vi "Read Status.vi"(8 "Error In":errorcluster, 11 "Writer In":refnum<class "Writer.lvclass">) -> (0 "Error Out":errorcluster, 2 "Status":T1, 3 "Writer Out":refnum<class "Writer.lvclass">)   [LabVIEW 2018, in "Toolkit.lvlib" / "Writer.lvclass"]
doc: "Gets the latest status of the internal encoder."
uses:
  Writer.lvclass
  Controls/Status.ctl
  Writer.lvclass/Writer.ctl
  Toolkit.lvlib
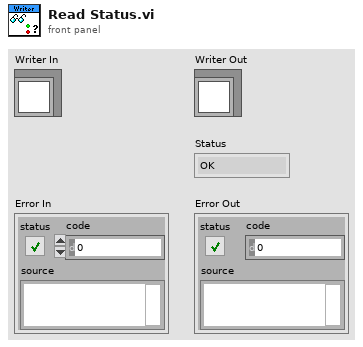
[diagram p1: front panel]
types:
  T1 = typedef "Toolkit.lvlib/Status.ctl" = enum32{"OK", "Out of Memory", "Null Value", "Encoder", "Decoder"}
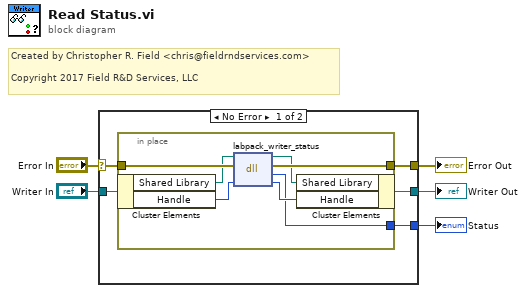
[diagram p0: block diagram]
diagram:
  # "Created by Christopher R. Field <chris@fieldrndservices.com>\n\nCopyright 2017 Field R&D Services, LLC"
  n1 = case shown="No Error" "Error In" {
    selector: "Error In" -> [w10 w18]
    tunnel: "Writer In" -> [w8 w19]
    tunnel: [w7 w19] -> w3
    tunnel: [w9 w18] -> w2
    tunnel: [w6 _] -> w1
    frame No Error {
      n2 = in-place {
        in-place-border: w10 -> [w17]
        in-place-border: [w16] -> w9
        in-place-border: [w11] -> w6
        n3 = in-place-cluster #1(w8) -> ("Shared Library"=w13:path, "Handle"=w15:u64)
        n4 = dll-call lib="D:/Users/cfield/Code/MessagePack/LabPack/LabVIEW/trunk/src/LabPack/Private/labpack-x64.dll" fn="labpack_writer_status"(path in=w13, error in=w17, "writer"=w15) -> (path out=w12:path, error out=w16:errorcluster, "return type"=w11:u32, "writer"=w14:u64)  [unwired: 1 in]
        n5 = in-place-cluster #1("Shared Library"=w12, "Handle"=w14) -> (w7:refnum<class "Writer.lvclass">)
      }
    }
    frame Error {
    }
  }
  "Writer Out" <- w3
  "Error Out" <- w2
  "Status" <- w1
